vi "FRCts20_Backend_TeamRoot_POST.vi"(6 "Message Attributes":T4, 8 "error in (no error)":errorcluster, 10 "Data":string, 11 "Engine_Refnums":T1) -> (0 "error out":errorcluster)   [LabVIEW 2014, in "FRCts20_Backend_Engine.lvlib"]
doc: "Creates a new team, called by the Team API. Expects all team data (number, name, etc.)"
uses:
  FRCts20_Backend_Engine.lvlib
  Dependencies/Keyed Array/KeyedArray.ctl
  FRCts20_Backend_EngineRefnums.ctl
  INI_Accessor/FRCts20_Backend_INI Controller.lvclass
  Dependencies/AMC/_SubVIs/TypeDefs/Message Queue.ctl
  Dependencies/AMC/_SubVIs/TypeDefs/Message.ctl
  <vilib>/addons/database/Connection.llb/Conn ObjectReference.ctl
  FRCts20_Backend_FGVOperation.ctl
  FRCts20_Backend_API/FRCts20_Backend_API_TeamRoot.ctl
  FRCts20_Backend_API/FRCts20_Backend_API_SW.ctl
  FRCts20_Backend_API/FRCts20_Backend_API.lvlib
  Dependencies/Keyed Array/Tools_KeyedArray.lvlib
  Dependencies/AMC/AMC.lvlib
  <vilib>/addons/database/NI_Database_API.lvlib
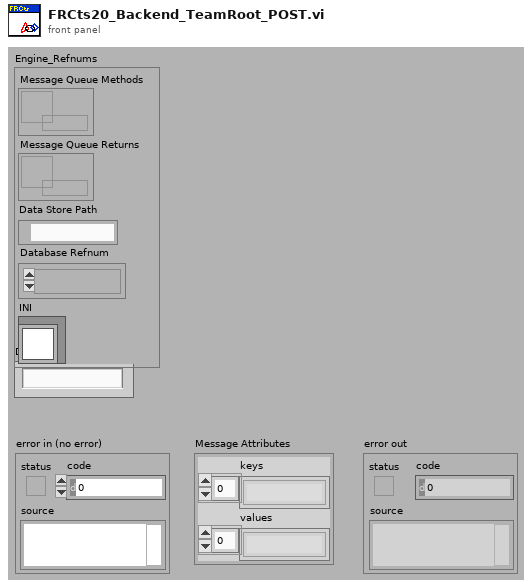
[diagram p1: front panel]
types:
  T1 = typedef "FRCts20_Backend_Engine.lvlib/FRCts20_Backend_EngineRefnums.ctl" = cluster{"Message Queue Methods":T2, "Message Queue Returns":T2, "Data Store Path":path, "Database Refnum":T3, "INI":refnum<class "FRCts20_Backend_INI Controller.lvclass">}
  T2 = typedef "AMC.lvlib/Message Queue.ctl" = refnum<queue>
  T3 = typedef "NI_Database_API.lvlib/Conn ObjectReference.ctl" = refnum<k1>
  T4 = typedef "Tools_KeyedArray.lvlib/KeyedArray.ctl" = cluster{"keys":string[], "values":string[]}
  T5 = typedef "FRCts20_Backend_Engine.lvlib/FRCts20_Backend_API.lvlib/FRCts20_Backend_API_TeamRoot.ctl" = cluster{"Teams":cluster{"Team Index":u32, "Team Number":u32, "Team ID":u32, "Team Name":string, "Short Team Name":string, "Nick Name":string, "Robot Name":string, "City":string, "State":string, "Country":string, "Rookie Year":u32, "SWType":T6, "CAN":bool, "Vision":bool, "Kinect":bool, "Tags":string, "Avatar":string, "Events":cluster{"EventIndex":u32, "EventName":string, "IsLive":bool}[]}[], "APIReturn":string}
  T6 = typedef "FRCts20_Backend_Engine.lvlib/FRCts20_Backend_API.lvlib/FRCts20_Backend_API_SW.ctl" = string
  T7 = typedef "FRCts20_Backend_Engine.lvlib/FRCts20_Backend_FGVOperation.ctl" = enum16{"Initialize", "EnqueueMessage", "EnqueueDataReturn", "FlushMessage", "FlushDataReturn"}
  T8 = cluster{"Team Index":u32, "Team Number":u32, "Team ID":u32, "Team Name":string, "Short Team Name":string, "Nick Name":string, "Robot Name":string, "City":string, "State":string, "Country":string, "Rookie Year":u32, "SWType":T6, "CAN":bool, "Vision":bool, "Kinect":bool, "Tags":string, "Avatar":string, "Events":cluster{"EventIndex":u32, "EventName":string, "IsLive":bool}[]}[]
  T9 = cluster{"Team Index":u32, "Team Number":u32, "Team ID":u32, "Team Name":string, "Short Team Name":string, "Nick Name":string, "Robot Name":string, "City":string, "State":string, "Country":string, "Rookie Year":u32, "SWType":T6, "CAN":bool, "Vision":bool, "Kinect":bool, "Tags":string, "Avatar":string, "Events":cluster{"EventIndex":u32, "EventName":string, "IsLive":bool}[]}
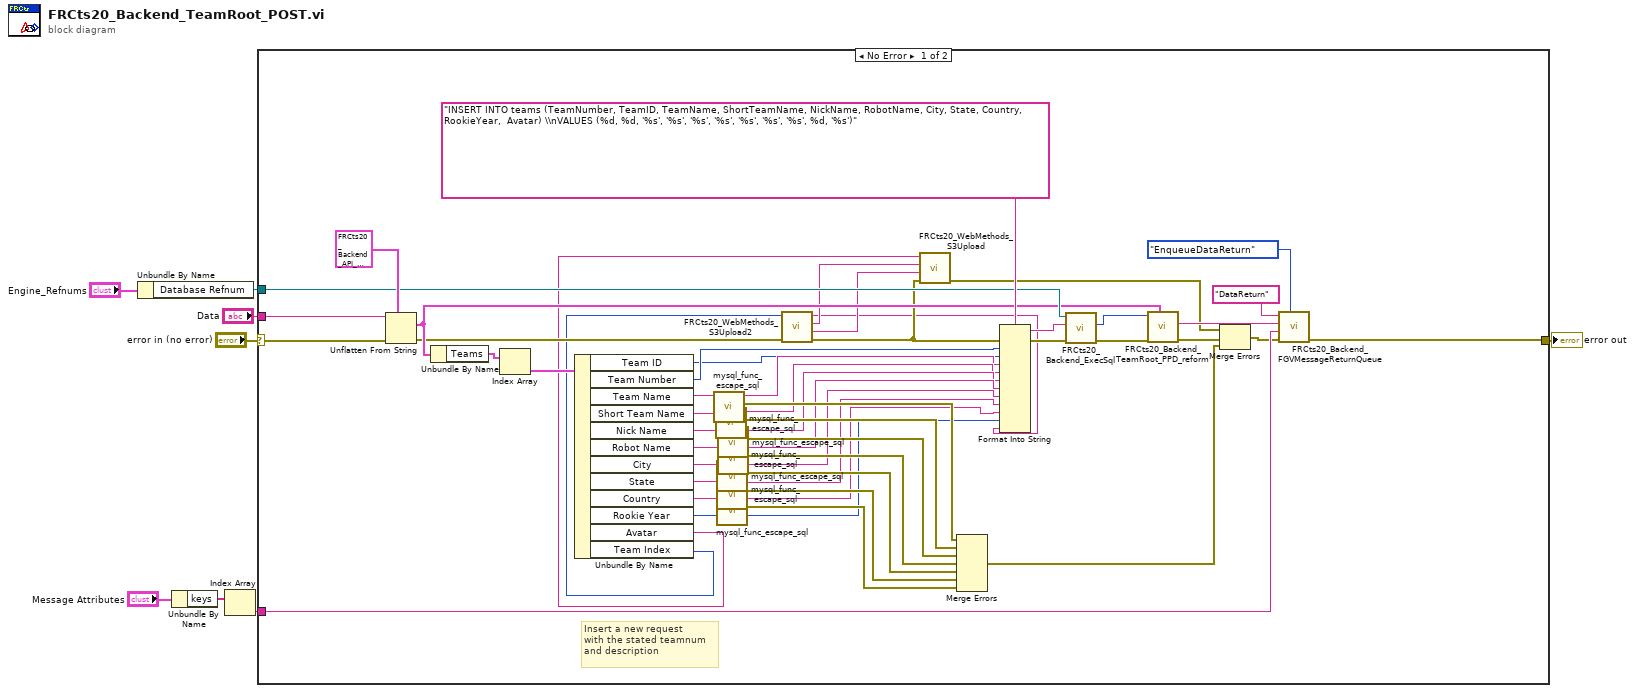
[diagram p0: block diagram]
diagram:
  n1 = Unbundle By Name("Engine_Refnums") -> ("Database Refnum"=w5:T3)
  n2 = Unbundle By Name("Message Attributes") -> ("keys"=w2:string[])
  n3 = Index Array(array=w2) -> (element=w1:string)  [unwired: 1 in]
  n4 = case shown="No Error" "error in (no error)" {
    selector: "error in (no error)" -> [w58 w61]
    tunnel: [w35 w61] -> w7
    tunnel: w5 -> [w53 _]
    tunnel: "Data" -> [w59 _]
    tunnel: w1 -> [w60 _]
    frame No Error {
      # "Insert a new request\nwith the stated teamnum\nand description"
      n5 = Unflatten From String(type=T5 {"Teams"=[{"Team Index"=0, "Team Number"=0, "Team ID"=0, "Team Name"="", "Short Team Name"="", "Nick Name"="", "Robot Name"="", "City"="", "State"="", "Country"="", "Rookie Year"=0, "SWType"="", "CAN"=FALSE, "Vision"=FALSE, "Kinect"=FALSE, "Tags"="", "Avatar"="", "Events"=[]}], "APIReturn"=""} ("Team Root"), binary string=w59, error in (no error)=w58) -> (value=w47:T5, error out=w41:errorcluster)  [unwired: 2 in, 1 out]
      n6 = Unbundle By Name(w47) -> ("Teams"=w46:T8)
      n7 = Index Array(array=w46) -> (element=w45:T9)  [unwired: 1 in]
      n8 = Unbundle By Name(w45) -> ("Team ID"=w9:u32, "Team Number"=w44:u32, "Team Name"=w33:string, "Short Team Name"=w32:string, "Nick Name"=w31:string, "Robot Name"=w30:string, "City"=w29:string, "State"=w28:string, "Country"=w27:string, "Rookie Year"=w17:u32, "Avatar"=w39:string, "Team Index"=w38:u32)
      n9 = call "mysql_func_escape_sql.vi"("sqlin"=w33) -> ("error out"=w26:errorcluster, "escaped"=w10:string)  [unwired: 9 in]
      n10 = call "mysql_func_escape_sql.vi"("sqlin"=w32) -> ("error out"=w25:errorcluster, "escaped"=w11:string)  [unwired: 9 in]
      n11 = call "mysql_func_escape_sql.vi"("sqlin"=w29) -> ("error out"=w22:errorcluster, "escaped"=w14:string)  [unwired: 9 in]
      n12 = call "mysql_func_escape_sql.vi"("sqlin"=w28) -> ("error out"=w21:errorcluster, "escaped"=w15:string)  [unwired: 9 in]
      n13 = call "mysql_func_escape_sql.vi"("sqlin"=w27) -> ("error out"=w20:errorcluster, "escaped"=w16:string)  [unwired: 9 in]
      n14 = call "mysql_func_escape_sql.vi"("sqlin"=w31) -> ("error out"=w24:errorcluster, "escaped"=w12:string)  [unwired: 9 in]
      n15 = call "mysql_func_escape_sql.vi"("sqlin"=w30) -> ("error out"=w23:errorcluster, "escaped"=w13:string)  [unwired: 9 in]
      n16 = call "FRCts20_WebMethods_S3Upload2.vi"("error in (no error)"=w41, "Team Index"=w38) -> ("error out"=w40:errorcluster, "Bucket"=w42:string, "Object Path"=w43:string, "S3 URL"=w18:string)  [unwired: 6 in]
      n17 = call "FRCts20_WebMethods_S3Upload.vi"("error in (no error)"=w40, "Bucket"=w42, "Object Path"=w43, "Temporary URL"=w39) -> ("error out"=w34:errorcluster)  [unwired: 7 in]
      n18 = Merge Errors(w26, w25, w24, w23, w22, w21, w20) -> (w19:errorcluster)
      n19 = Format Into String(format string="INSERT INTO teams (TeamNumber, TeamID, TeamName, ShortTeamName, NickName, RobotName, City, State, Country, RookieYear,  Avatar) \\nVALUES (%d, %d, '%s', '%s', '%s', '%s', '%s', '%s', '%s', %d, '%s')", error in=w40, w44, w9, w10, w11, w12, w13, w14, w15, w16, w17, w18) -> (resulting string=w48:string, error out=w52:errorcluster)  [unwired: 1 in]
      n20 = call "FRCts20_Backend_ExecSql.vi"("error in (no error)"=w52, "format string"=w48, "Refnum in"=w53) -> ("error out"=w50:errorcluster, "rows affected"=w51:i32)  [unwired: 6 in, 1 out]
      n21 = call "FRCts20_Backend_TeamRoot_PPD_reform.vi"("Team Root"=w47, "error in (no error)"=w50, "rows affected"=w51) -> ("error out"=w37:errorcluster, "data string"=w49:string)  [unwired: 7 in]
      n22 = Merge Errors(w34, w37, w19) -> (w36:errorcluster)
      n23 = call "FRCts20_Backend_FGVMessageReturnQueue.vi"("Operation"=FRCts20_Backend_FGVOperation."EnqueueDataReturn", "error in (no error)"=w36, "Key"=w60, "Message Value"=w49, "Message Name"="DataReturn") -> ("error out"=w35:errorcluster)  [unwired: 5 in, 1 out]
    }
    frame Error {
    }
  }
  "error out" <- w7
